vi "lOOK AT NANOVNA.vi"() -> ()   [LabVIEW 2020]
uses:
  common/record_file_handler/VFH-VNA_File_Handler.lvlib
panel:
  out "Cluster":T1 {"Z''" format="%#_5p"; "Z'" format="%#_5p"; "|Z|" format="%#_5p"; "Loss" format="%#_5p"; "Deg" format="%#_5p"; "Phi" format="%#_5p"; "Mag" format="%#_5p"; "S11 I" format="%#_5p"; "S11 R" format="%#_5p"}
  out "Array":dbl[](array[numeric]) format="%#_5p"
  out "Freq":dbl format="%#_6p"
  in  "index":i32
  in  "Stop":bool
  in  "Folder Path":path=path "C:/NanoVNA-App/Recordings/2024-07-26 09-29-22"
  in  "Tab Control":enum32{"Page 1", "Page 2"}(tab)
  out "Complex":cluster{"Frequency":dbl[], "S21_Imag":dbl[]}[](graph)
  in  "Log Raw":bool
  out "Calc":cluster{"Frequency":dbl[], "S11_Imag":dbl[]}[](graph)
  out "Raw":cluster{"Frequency":dbl[], "S21_Imag":dbl[]}[](graph)
  in  "Log calc":bool
  in  "Log complex":bool
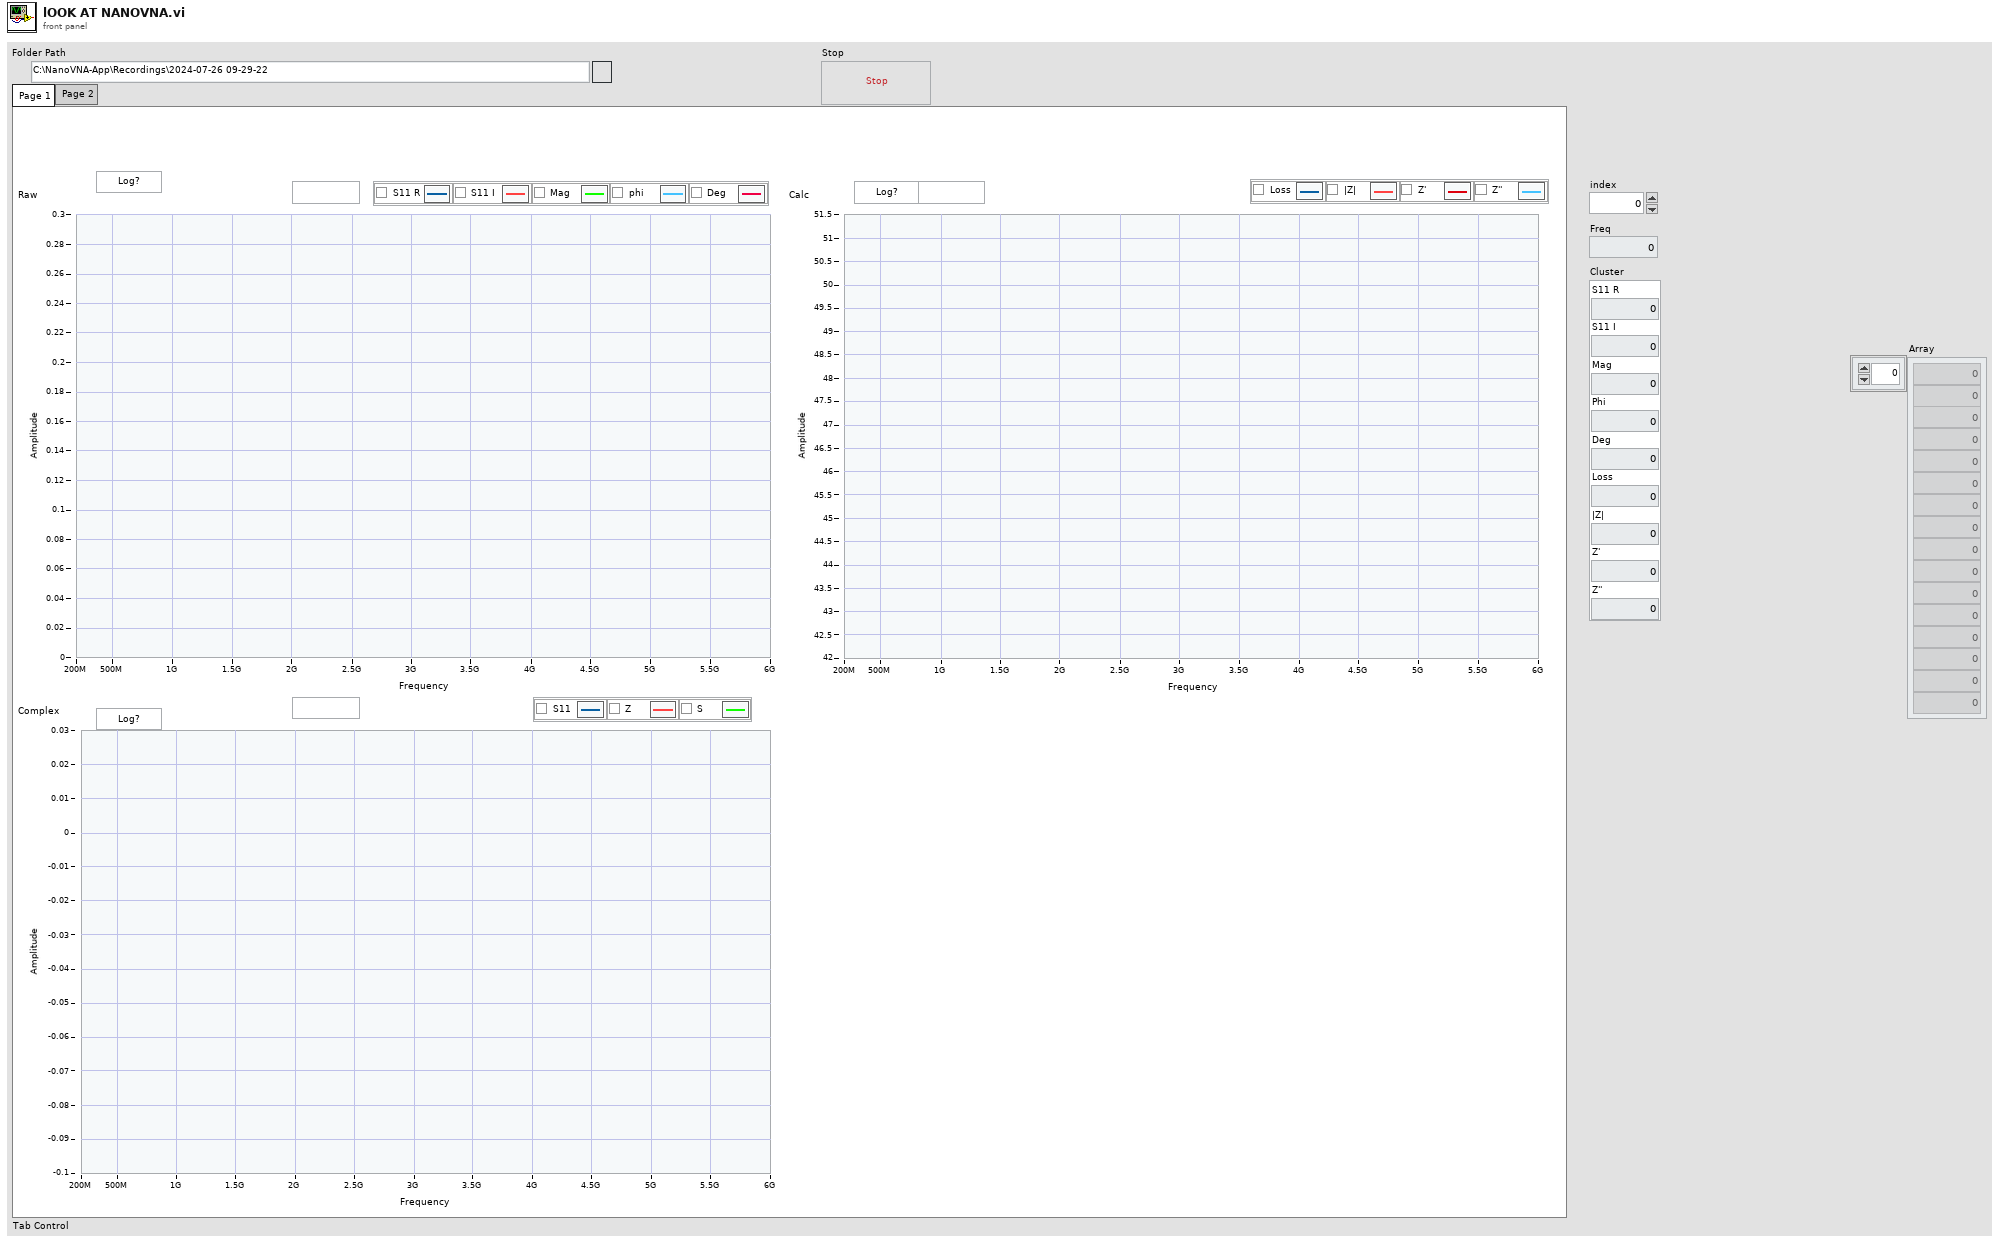
[diagram p1: front panel]
types:
  T1 = cluster{"S11 R":dbl, "S11 I":dbl, "Mag":dbl, "Phi":dbl, "Deg":dbl, "Loss":dbl, "|Z|":dbl, "Z'":dbl, "Z''":dbl}
  T2 = typedef "VFH-VNA_File_Handler.lvlib/VFH-file_cluster-NanoVNA.ctl" = cluster{"Frequency":dbl[], "S11_Real":dbl[], "S11_Imag":dbl[], "S21_Real":dbl[], "S21_Imag":dbl[], "S12_Real":dbl[], "S12_Imag":dbl[], "S22_Real":dbl[], "S22_Imag":dbl[]}
  T3 = cluster{"Complex Input":cluster{"Frequency":dbl[], "Array":cdb[]}, "Complex Z":cluster{"Frequency":dbl[], "Array":cdb[]}, "Complex S":cluster{"Frequency":dbl[], "Array":cdb[]}}
  T4 = cluster{"Loss":cluster{"Frequency":dbl[], "Array":dbl[]}, "Z Modulus":cluster{"Frequency":dbl[], "Array":dbl[]}, "Z'":cluster{"Frequency":dbl[], "Array":dbl[]}, "Z''":cluster{"Frequency":dbl[], "Array":dbl[]}}
  T5 = cluster{"S11'":cluster{"Frequency":dbl[], "S11_Real":dbl[]}, "S11''":cluster{"Frequency":dbl[], "S11_Real":dbl[]}, "Magnitude":cluster{"Frequency":dbl[], "Array":dbl[]}, "Eta":cluster{"Frequency":dbl[], "Array":dbl[]}, "Phase":cluster{"Frequency":dbl[], "Array":dbl[]}}
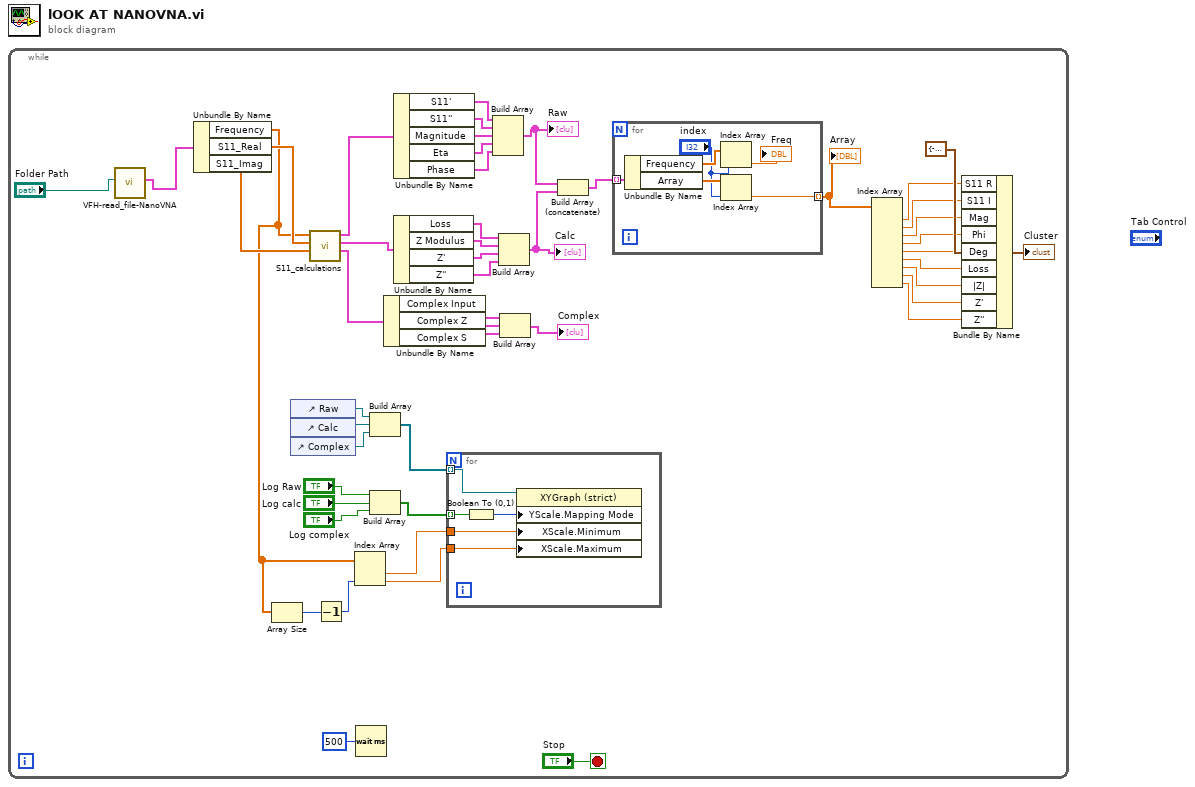
[diagram p0: block diagram]
diagram:
  n1 = while {
    stop <- "Stop" stop-if-true
    n2 = call "VFH-read_file-NanoVNA.vi"("file path (dialog if empty)"="Folder Path") -> ("output cluster"=w8:T2)  [unwired: 9 in, 1 out]
    n3 = Unbundle By Name(w8) -> ("Frequency"=w3:dbl[], "S11_Real"=w6:dbl[], "S11_Imag"=w5:dbl[])
    n4 = Array Size(array=w3) -> (size(s)=w4:i32)
    n5 = control-ref of="Raw"() -> (w17:refnum<vi>)
    n6 = control-ref of="Calc"() -> (w16:refnum<vi>)
    n7 = control-ref of="Complex"() -> (w15:refnum<vi>)
    n8 = call "S11_calculations.vi"("S11_Imag"=w5, "S11_Real"=w6, "Frequency"=w3) -> ("Complex"=w34:T3, "Calc"=w44:T4, "Raw"=w50:T5)  [unwired: 6 in]
    n9 = Decrement(x=w4) -> (x-1=w2:i32)
    n10 = Index Array(array=w3, index #2=w2) -> (element #1=w9:dbl, element #2=w1:dbl)  [unwired: 1 in]
    n11 = Wait (ms)(milliseconds to wait=u32 500) -> ()  [unwired: 1 out]
    n12 = Build Array(w17, w16, w15) -> (w14:refnum<vi>[])
    n13 = Build Array("Log Raw", "Log calc", "Log complex") -> (w10:bool[])
    n14 = Unbundle By Name(w34) -> ("Complex Input"=w35:cluster{"Frequency":dbl[], "Array":cdb[]}, "Complex Z"=w36:cluster{"Frequency":dbl[], "Array":cdb[]}, "Complex S"=w37:cluster{"Frequency":dbl[], "Array":cdb[]})
    n15 = Unbundle By Name(w50) -> ("S11'"=w49:cluster{"Frequency":dbl[], "S11_Real":dbl[]}, "S11''"=w48:cluster{"Frequency":dbl[], "S11_Real":dbl[]}, "Magnitude"=w47:cluster{"Frequency":dbl[], "Array":dbl[]}, "Eta"=w46:cluster{"Frequency":dbl[], "Array":dbl[]}, "Phase"=w45:cluster{"Frequency":dbl[], "Array":dbl[]})
    n16 = Unbundle By Name(w44) -> ("Loss"=w43:cluster{"Frequency":dbl[], "Array":dbl[]}, "Z Modulus"=w42:cluster{"Frequency":dbl[], "Array":dbl[]}, "Z'"=w41:cluster{"Frequency":dbl[], "Array":dbl[]}, "Z''"=w40:cluster{"Frequency":dbl[], "Array":dbl[]})
    n17 = for {
      tunnel: w14 -> [w55] mode=indexing
      tunnel: w10 -> [w54] mode=indexing
      tunnel: w9 -> [w52]
      tunnel: w1 -> [w51]
      n18 = Boolean To (0,1)(Boolean=w54) -> (0, 1=w53:i16)
      n19 = property class="XYGraph (strict)"(reference=w55, "YScale.Mapping Mode"=w53, "XScale.Minimum"=w52, "XScale.Maximum"=w51) -> ()  [unwired: 1 in, 2 out]
    }
    n20 = Build Array(w49, w48, w47, w46, w45) -> (w31:cluster{"Frequency":dbl[], "Array":dbl[]}[])
    "Raw" <- w31
    n21 = Build Array(w43, w42, w41, w40) -> (w32:cluster{"Frequency":dbl[], "Array":dbl[]}[])
    "Calc" <- w32
    n22 = Build Array(w35, w36, w37) -> (→"Complex":cluster{"Frequency":dbl[], "Array":cdb[]}[])
    n23 = Build Array (concatenate)(w31, w32) -> (w30:cluster{"Frequency":dbl[], "Array":dbl[]}[])
    n24 = for {
      tunnel: w30 -> [w61] mode=indexing
      tunnel: [w56] -> w29 mode=indexing
      n25 = Unbundle By Name(w61) -> ("Frequency"=w59:dbl[], "Array"=w60:dbl[])
      n26 = Index Array(array=w59, index="index") -> (element=→"Freq":dbl)
      n27 = Index Array(array=w60, index="index") -> (element=w56:dbl)
    }
    "Array" <- w29
    n28 = Index Array(array=w29) -> (element #1=w26:dbl, element #2=w25:dbl, element #3=w24:dbl, element #4=w23:dbl, element #5=w22:dbl, element #6=w21:dbl, element #7=w20:dbl, element #8=w19:dbl, element #9=w18:dbl)  [unwired: 9 in]
    n29 = Bundle By Name(cluster=T1 {"S11 R"=-0.13079270605384616, "S11 I"=-0.13079270605384616, "Mag"=-0.13079270605384616, "Phi"=-0.13079270605384616, "Deg"=-0.13079270605384616, "Loss"=-0.13079270605384616, "|Z|"=-0.13079270605384616, "Z'"=-0.13079270605384616, "Z''"=-0.13079270605384616} ("Cluster"), "S11 R"=w26, "S11 I"=w25, "Mag"=w24, "Phi"=w23, "Deg"=w22, "Loss"=w21, "|Z|"=w20, "Z'"=w19, "Z''"=w18) -> (→"Cluster":T1)
  }
